vi "Ctor.vi"(8 "error in (no error)":errorcluster) -> (0 "error out":errorcluster, 3 "HAL Manager out":refnum<class "HAL Manager.lvclass">)   [LabVIEW 2020, in "HAL.lvlib" / "HAL Manager.lvclass"]
uses:
  HAL Manager.lvclass
  Ref Data.ctl
  Device/Device.lvclass
  HAL Manager.lvclass/HAL Manager.ctl
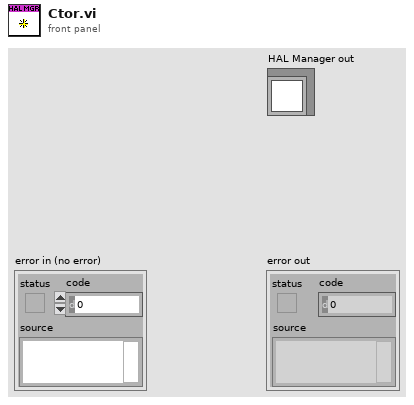
[diagram p1: front panel]
types:
  T1 = typedef "HAL.lvlib/HAL Manager.lvclass/Ref Data.ctl" = cluster{"Devices":refnum<class "Device.lvclass">[], "Type":string[], "Models":string[], "Name":string[]}
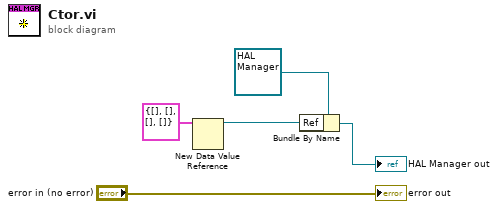
[diagram p0: block diagram]
diagram:
  n1 = New Data Value Reference(data value=T1 {"Devices"=[], "Type"=[], "Models"=[], "Name"=[]} ("Ref Data")) -> (data value reference=w1:refnum<data-value>)  [unwired: 1 in, 1 out]
  n2 = Bundle By Name(cluster=refnum<class "HAL Manager.lvclass"> refnum ("HAL Manager in"), "Ref"=w1) -> (→"HAL Manager out":refnum<class "HAL Manager.lvclass">)
  "error out" <- "error in (no error)"
